vi "close_TCP.vi"(4 "error in":errorcluster, 7 "connection ID":refnum<k5>) -> (0 "error out":errorcluster)   [LabVIEW 2016, in "AMC_VIs.lvlib"]
doc: "Initializes and connects the selected ECC (0..n).\nThis has to be done before any other function (except ECC_Check and ECC_ReleaseInfo) can be called.\nThe returned handle is used to address the device in further communication.\n\nInput\n deviceNo* index of the device to connect (0..n)\n error error message\n\nOutput\n deviceHandle device handle\n error error message\n\n* required inputs"
uses:
  AMC_VIs.lvlib
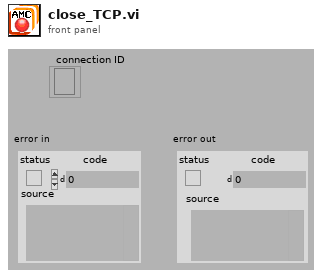
[diagram p1: front panel]
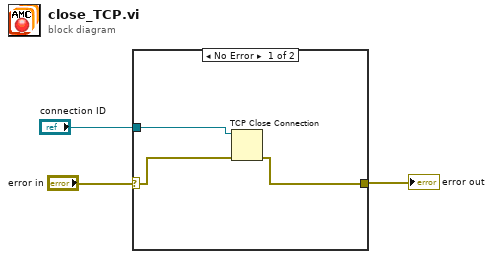
[diagram p0: block diagram]
diagram:
  n1 = case shown="No Error" "error in" {
    selector: "error in" -> [w5 w7]
    tunnel: [w4 w7] -> w2
    tunnel: "connection ID" -> [w6 _]
    frame No Error {
      n2 = TCP Close Connection(connection ID=w6, error in (no error)=w5) -> (error out=w4:errorcluster)  [unwired: 1 in, 1 out]
    }
    frame Error {
    }
  }
  "error out" <- w2
